vi "WPI_SafetyOutputEngine.vi"   [LabVIEW 2017]
doc: "This calls each registered Safety Test VI. It uses the Call By Reference Node which requires strictly typed references. The Call By Reference Node is used because strictly typed references preload everything so the call is fast. The regular VI Run method was too slow."
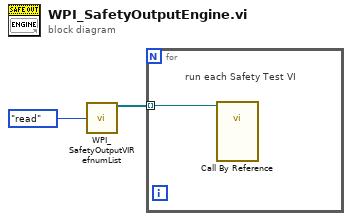
[diagram p0: block diagram]
diagram:
  n1 = call <vilib>:"WPI_SafetyOutputVIRefnumList.vi"("menu"=enum16{"read", "add", "remove"}."read") -> ("VI Refnums"=w1:refnum<vi>[])  [unwired: 1 in, 13 out]
  n2 = for {
    tunnel: w1 -> [w3] mode=indexing
    # "run each Safety Test VI"
    n3 = call-by-ref "?"(reference=w3) -> ()  [unwired: 2 in, 2 out]
  }
